vi "ConvertTargetPlatformToOperatingSystem.vi"(11 "Platform":T1) -> (3 "Operating System":string)   [LabVIEW 2016, in "VeriStandTestUtilities.lvlib"]
uses:
  VeriStandTestUtilities.lvlib
  TargetPlatform.ctl
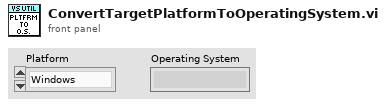
[diagram p1: front panel]
types:
  T1 = typedef "VeriStandTestUtilities.lvlib/TargetPlatform.ctl" = enum16{"Windows", "Linux64CRIO", "Linux64PXI", "LinuxARM", "PharLap"}
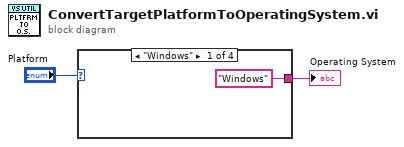
[diagram p0: block diagram]
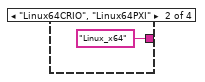
[diagram p2: hidden frame]
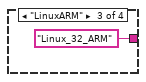
[diagram p3: hidden frame]
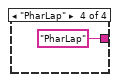
[diagram p4: hidden frame]
diagram:
  n1 = case shown="\"Windows\"" "Platform" {
    tunnel: ["Windows" "Linux_x64" "Linux_32_ARM" "PharLap"] -> w2
    frame "Windows" {
    }
    frame "Linux64CRIO", "Linux64PXI" {
    }
    frame "LinuxARM" {
    }
    frame "PharLap" {
    }
  }
  "Operating System" <- w2
